vi "Configure Temperature.vi"   [LabVIEW 2021, in "Agilent 34420.lvlib"]
doc: "Configures specific temperature settings."
uses:
  <instrlib>/Agilent 34420/Agilent 34420.lvlib
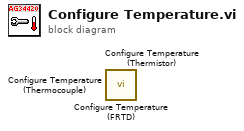
[diagram p0: block diagram]
diagram:
  n1 = call <instrlib>:"Configure Temperature (FRTD).vi"() -> ()  [unwired: 14 in, 2 out]
  n2 = call <instrlib>:"Configure Temperature (Thermistor).vi"() -> ()  [unwired: 14 in, 2 out]
  n3 = call <instrlib>:"Configure Temperature (Thermocouple).vi"() -> ()  [unwired: 14 in, 2 out]
